vi "GUI_Cameras.vi"() -> ()   [LabVIEW 2009]
panel:
  out "Array":string[](array[string])
  out "Class Name":string
  out "appended array":refnum<vi>[](array[refnum])
  out "array":string[][](array[string])
  in  "Data String":string
  in  "time to wait":i32=100
  out "block device port":bool
  out "block slow port":bool
  out "new Slow Data":bool
  out "new Device Data":bool
  in  "Tab Control 2":enum32{"debug", "plain", "plain 2"}(tab)
  out "message from device":string
  out "data out 2":string
  out "error out 3":errorcluster
  in  "after substring 3":string
  out "settings 2":string[][](array[string])=[["no error", ">>on"]]
  out "after substring 2":string="no error,>>on"
  in  "Tab Control":enum32{"Main", "Network settings", "internal"}(tab)
  in  "getSettings":bool
  in  "setTrigger":bool
  in  "String":string="subscribe>>image"
  in  "sent":bool
  in  "setSave":bool
  out "save":bool
  in  "setExposure":dbl=2.0
  out "exposure":dbl=2.0
  out "value":string
  out "trigger":bool
  out "Image Pixels (U8) 5":u8[][](graph)
  out "gain":dbl=2.0
  in  "setGain":dbl=2.0
  in  "local Port":u16=61557
  in  "Remote Host":string="192.168.10.156"
  in  "port or service name":u16=65533
  in  "timeout ms (100)":i32=500
  out "fast ID":refnum<k16>
  out "slow ID":refnum<k16>
  out "error out":errorcluster
  in  "stop":bool
  # "61525"
  # "65535"
  # "61533"
  # "localhost"
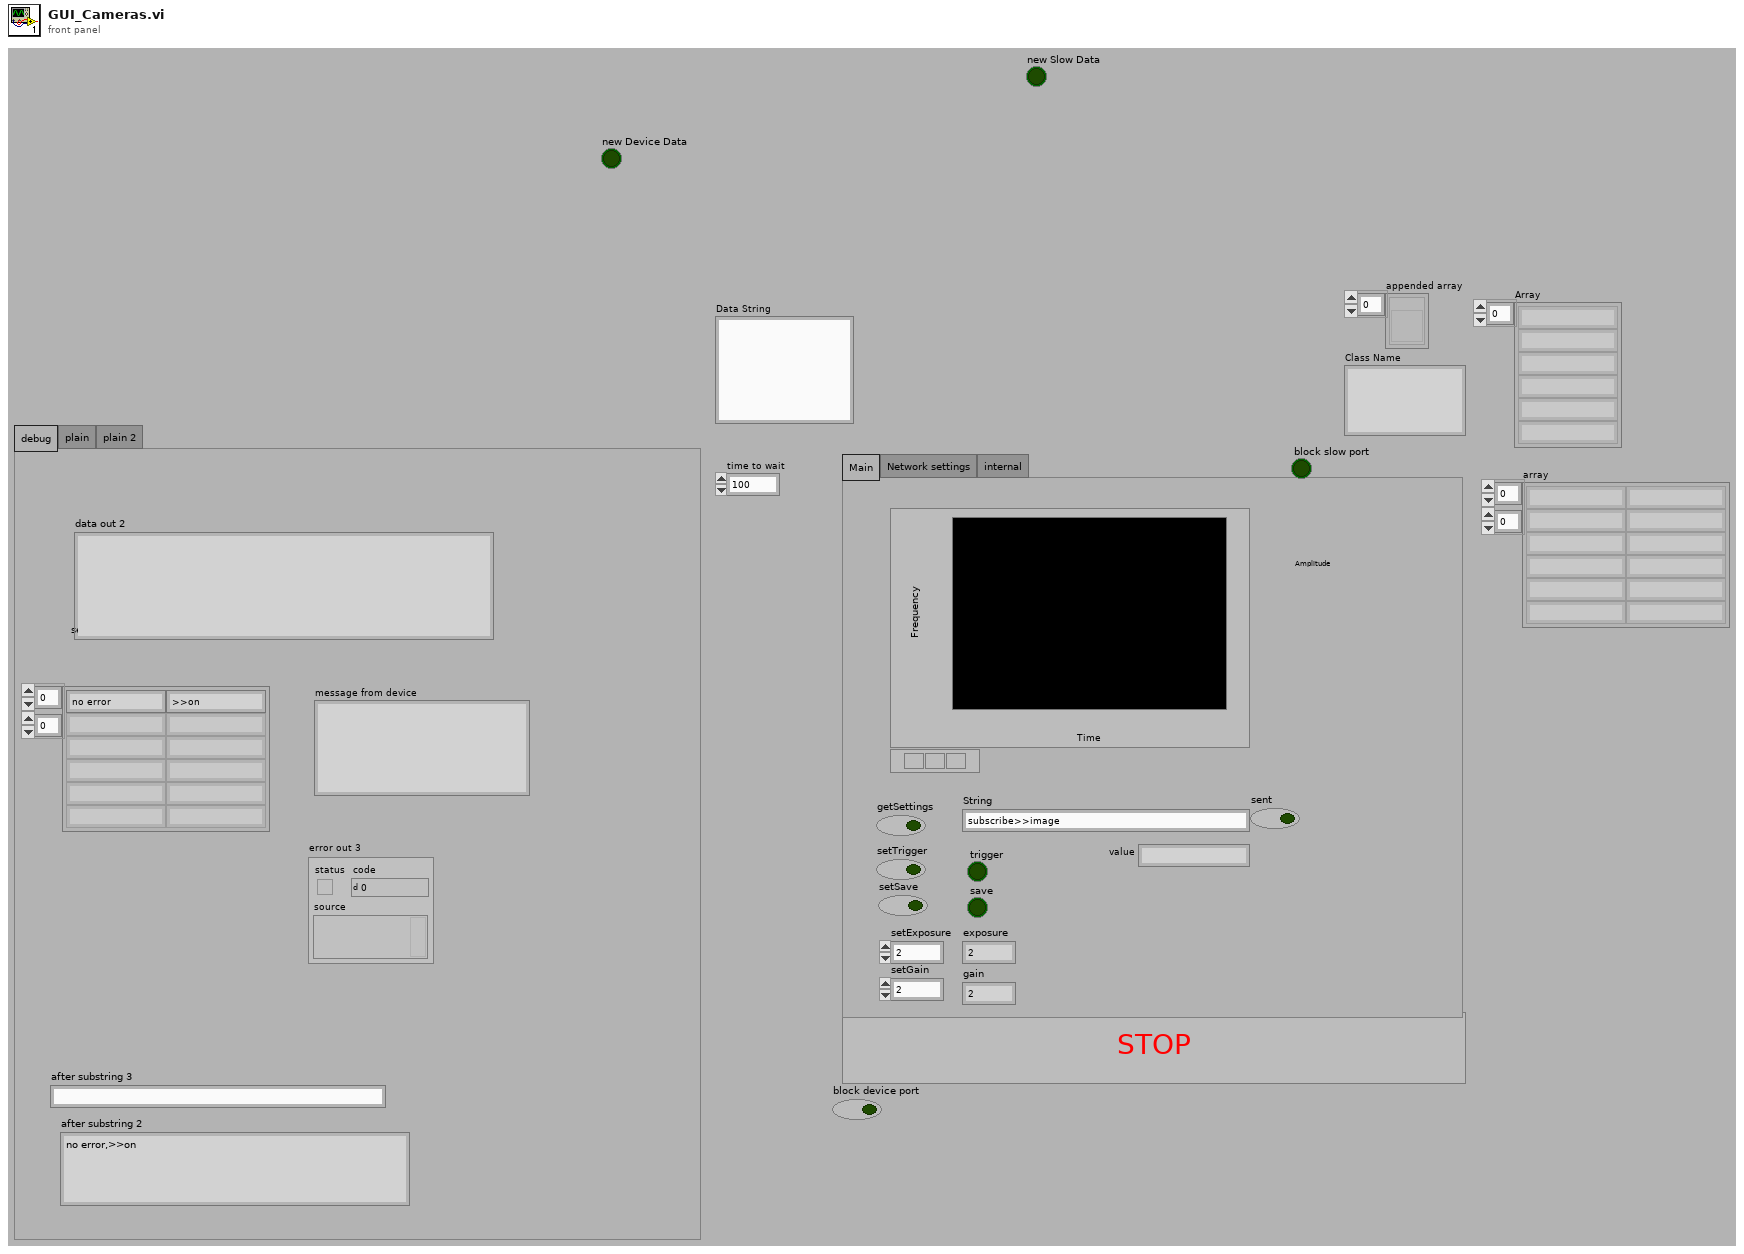
[diagram p1: front panel]
types:
  T1 = typedef "Image Type" = u32
  T2 = typedef "IMAQ Image.ctl" = refnum<image>
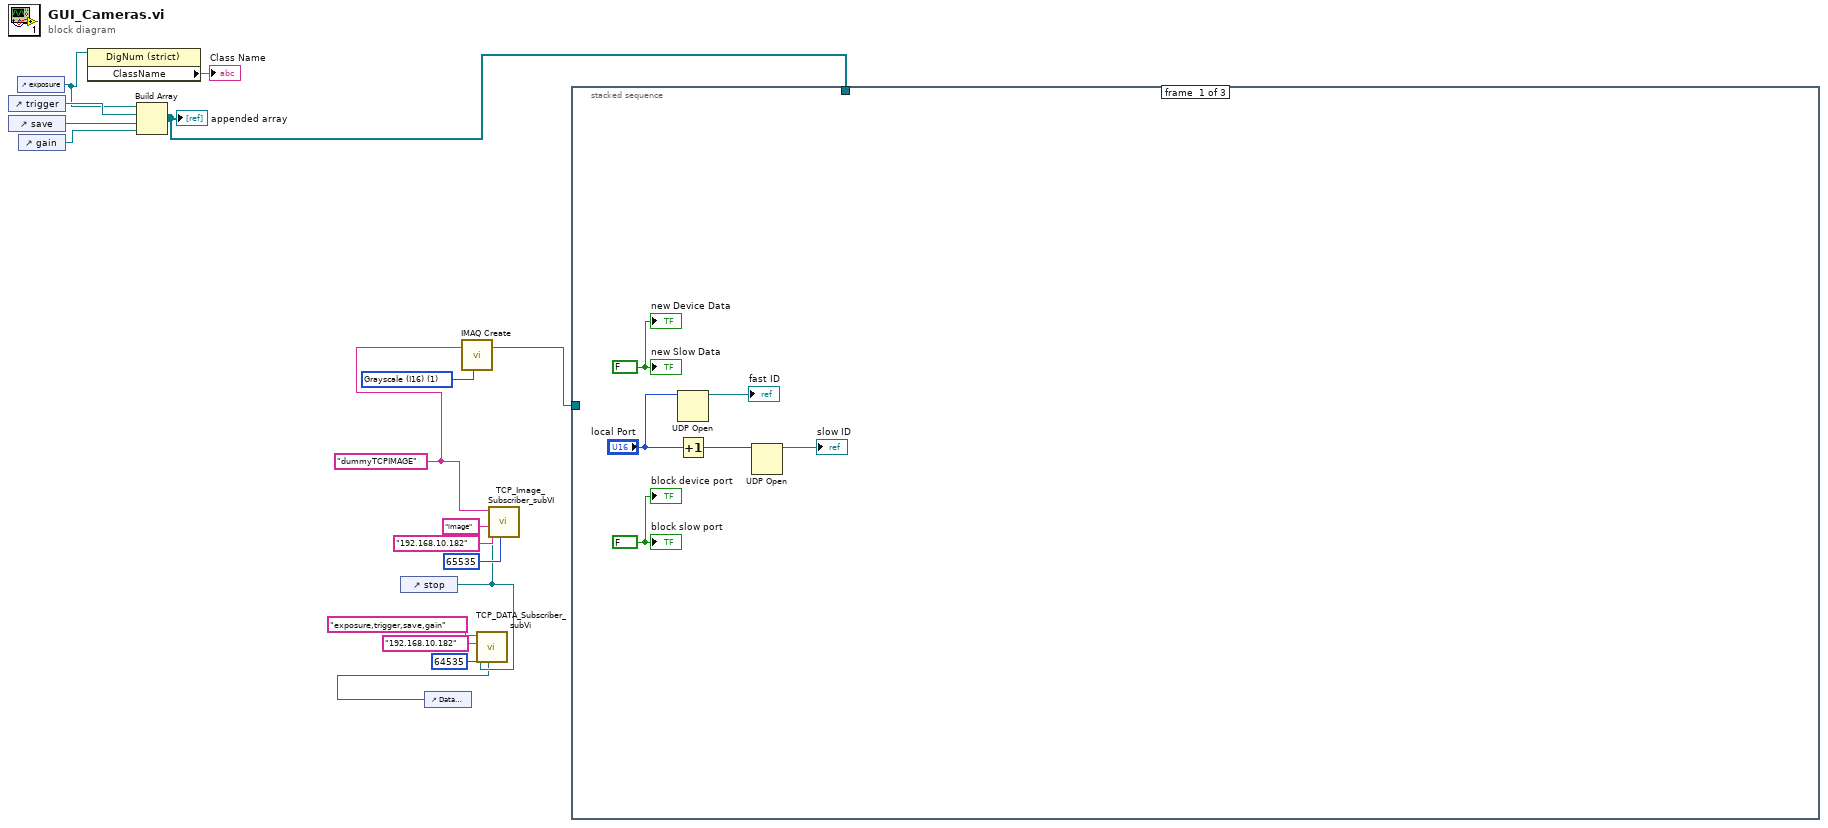
[diagram p0: block diagram]
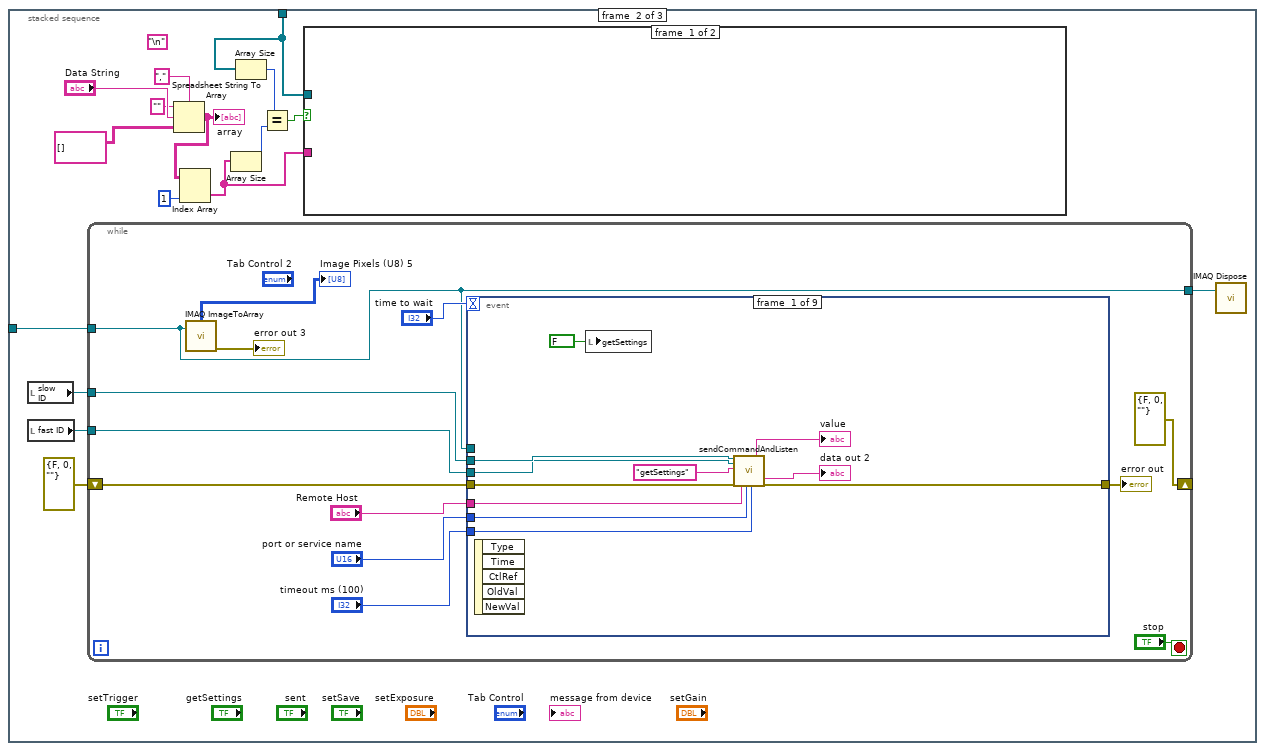
[diagram p2: hidden frame]
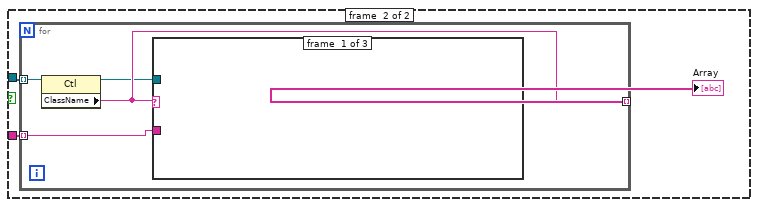
[diagram p3: hidden frame]
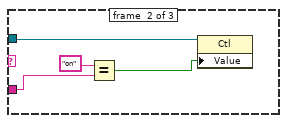
[diagram p4: hidden frame]
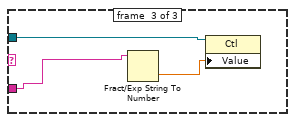
[diagram p5: hidden frame]
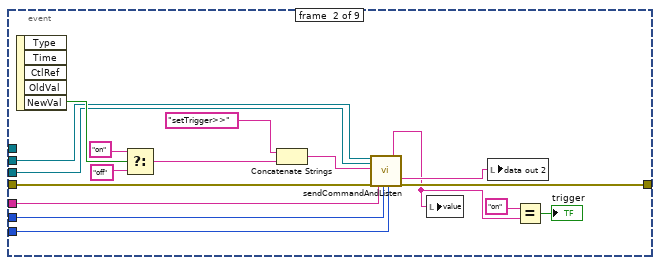
[diagram p6: hidden frame]
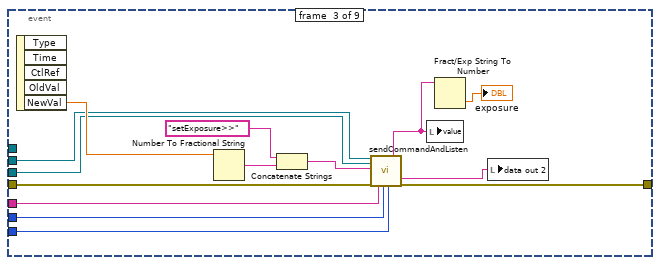
[diagram p7: hidden frame]
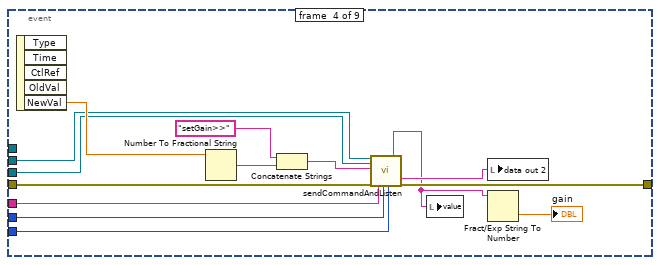
[diagram p8: hidden frame]
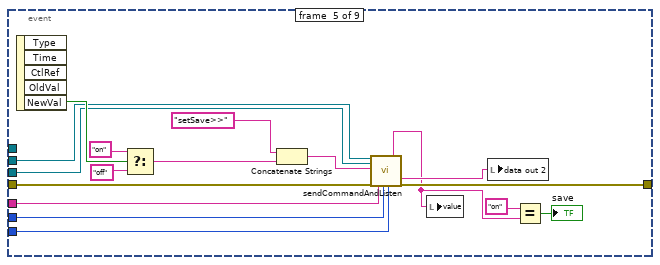
[diagram p9: hidden frame]
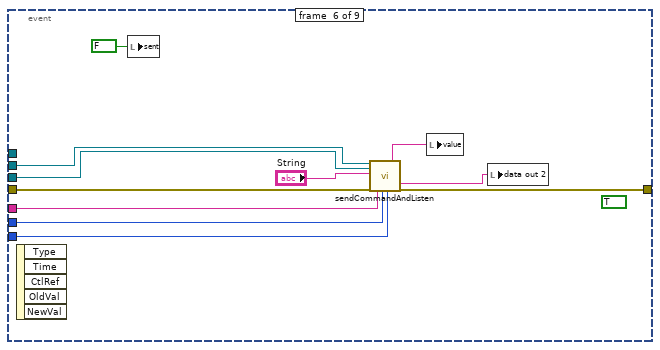
[diagram p10: hidden frame]
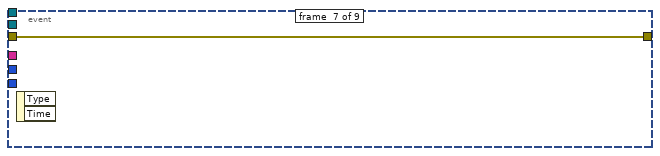
[diagram p11: hidden frame]
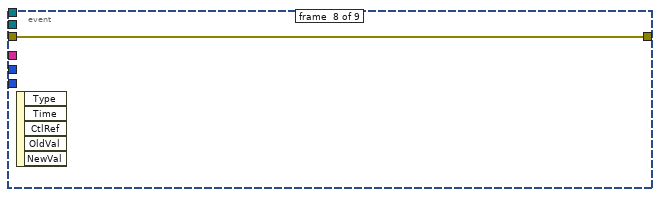
[diagram p12: hidden frame]
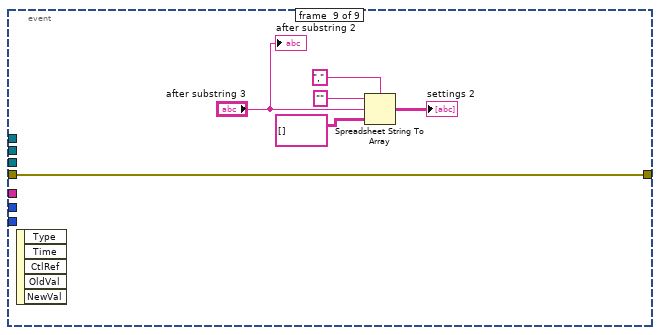
[diagram p13: hidden frame]
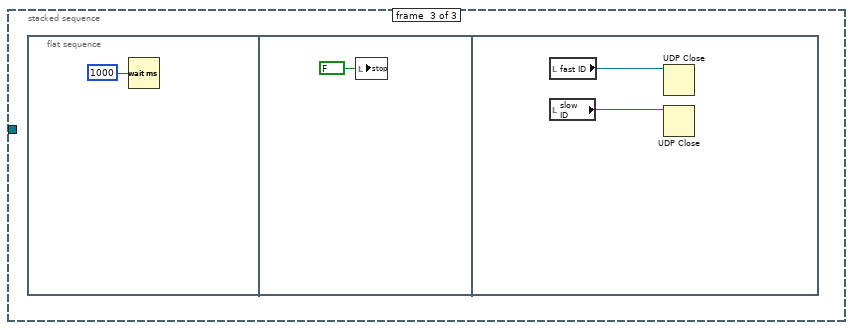
[diagram p14: hidden frame]
diagram:
  w12 = "dummyTCPIMAGE" ("Image Name")
  w17 = T1 1 items=["Grayscale (U8)", "Grayscale (I16)", "Grayscale (SGL)", "Complex (CSG)", "RGB (U32)", "HSL (U32)", "RGB (U64)", "Grayscale (U16)"] ("Image Type")
  n1 = control-ref of="trigger"() -> (w6:refnum<vi>)
  n2 = control-ref of="save"() -> (w5:refnum<vi>)
  n3 = control-ref of="exposure"() -> (w3:refnum<vi>)
  n4 = control-ref of="gain"() -> (w4:refnum<vi>)
  n5 = property class="DigNum (strict)"(reference=w3) -> ("ClassName"=→"Class Name":string)  [unwired: 1 in, 2 out]
  n6 = Build Array(w3, w6, w5, w4) -> (w1:refnum<vi>[])
  "appended array" <- w1
  n7 = control-ref of="stop"() -> (w8:refnum<vi>)
  n8 = control-ref of="Data String"() -> (w7:refnum<vi>)
  n9 = call "IMAQ Create"("Image Name"=w12, "Image Type"=w17) -> ("New Image"=w16:T2)  [unwired: 3 in, 1 out]
  n10 = call "TCP_DATA_Subscriber_subVi.vi"("data String"=w7, "stop 2"=w8, "Port"=u16 64535, "Machine"="192.168.10.182", "Subscriber list"="exposure,trigger,save,gain") -> ()  [unwired: 7 in]
  n11 = call "TCP_Image_Subscriber_subVI.vi"("Port"=u16 65535, "STOP"=w8, "Machine"="192.168.10.182", "subscriber list"="image", "Image Name"=w12) -> ()  [unwired: 7 in]
  n12 = stacked-sequence {
    tunnel: w16 -> [_ w36 _]
    tunnel: w1 -> [_ w30 _]
    frame #0 {
      w18 = FALSE ("new Device Data")
      w19 = FALSE
      n13 = UDP Open(11:"local Port") -> (port=→"fast ID":refnum<k16>)  [unwired: 4 in, 2 out]
      n14 = Increment(x="local Port") -> (x+1=w21:u16)
      n15 = UDP Open(11:w21) -> (port=→"slow ID":refnum<k16>)  [unwired: 4 in, 2 out]
      "block device port" <- w19
      "block slow port" <- w19
      "new Device Data" <- w18
      "new Slow Data" <- w18
    }
    frame #1 {
      (unwired) "\n"
      n16 = local read "slow ID"() -> (w37:refnum<k16>)
      n17 = local read "fast ID"() -> (w38:refnum<k16>)
      n18 = while {
        tunnel: w38 -> [w65]
        shift-right: [errorcluster {"status"=FALSE, "code"=0, "source"=""} ("error out")] -> _
        shift-left: errorcluster {"status"=FALSE, "code"=0, "source"=""} ("error out") -> [w63]
        tunnel: w37 -> [w57]
        tunnel: w36 -> [w54]
        tunnel: [w54] -> w35
        stop <- "stop" stop-if-true
        n19 = call "IMAQ ImageToArray"("Image"=w54) -> ("error out"=→"error out 3":errorcluster, "Image Pixels (U8)"=→"Image Pixels (U8) 5":u8[][])  [unwired: 3 in, 3 out]
        n20 = event shown="[2] \"setExposure\": Value Change" {
          selector: _ -> [_ _ _ _ _ _ _ _ _]
          dyn-events: _ -> [_ _ _ _ _ _ _ _ _]
          timeout: "time to wait" -> [_ _ _ _ _ _ _ _ _]
          tunnel: w65 -> [w74 w84 w103 w117 w132 w147 _ _ _]
          tunnel: [w72 w82 w101 w115 w129 w145 w151 w152 w158] -> w64
          tunnel: w63 -> [w73 w83 w102 w116 w130 w146 w151 w152 w158]
          tunnel: "Remote Host" -> [w71 w87 w99 w113 w133 w144 _ _ _]
          tunnel: "port or service name" -> [w70 w88 w98 w112 w128 w143 _ _ _]
          tunnel: "timeout ms (100)" -> [w69 w89 w97 w111 w127 w142 _ _ _]
          tunnel: w57 -> [w75 w85 w104 w118 w131 w148 _ _ _]
          tunnel: w54 -> [_ _ _ _ _ _ _ _ _]
          event #0 {
            n21 = event-data() -> ()  [unwired: 1 in, 5 out]
            n22 = local write "getSettings"(FALSE ("getSettings")) -> ()
            n23 = call "sendCommandAndListen.vi"("ID slow"=w75, "ID fast"=w74, "command in"="getSettings" ("data in"), "error in"=w73, "Remote Host"=w71, "port or service name"=w70, "timeout ms (100)"=w69) -> ("value"=→"value":string, "data out"=→"data out 2":string, "error out"=w72:errorcluster)  [unwired: 7 in, 3 out]
          }
          event #1 {
            n24 = event-data() -> ("NewVal"=w94:bool)  [unwired: 1 in, 4 out]
            n25 = Select(t="on", s=w94, f="off") -> (s? t:f=w90:string)
            n26 = Concatenate Strings("setTrigger>>" ("data in"), w90) -> (w86:string)
            n27 = call "sendCommandAndListen.vi"("ID slow"=w85, "ID fast"=w84, "command in"=w86, "error in"=w83, "Remote Host"=w87, "port or service name"=w88, "timeout ms (100)"=w89) -> ("value"=w79:string, "data out"=w81:string, "error out"=w82:errorcluster)  [unwired: 7 in, 3 out]
            n28 = local write "value"(w79) -> ()
            n29 = local write "data out 2"(w81) -> ()
            n30 = Equal?(x="on", y=w79) -> (x = y?=→"trigger":bool)
          }
          event #2 {
            n31 = event-data() -> ("NewVal"=w106:dbl)  [unwired: 1 in, 4 out]
            n32 = Number To Fractional String(number=w106) -> (F-format string=w107:string)  [unwired: 3 in]
            n33 = Concatenate Strings("setExposure>>" ("data in"), w107) -> (w105:string)
            n34 = call "sendCommandAndListen.vi"("ID slow"=w104, "ID fast"=w103, "command in"=w105, "error in"=w102, "Remote Host"=w99, "port or service name"=w98, "timeout ms (100)"=w97) -> ("value"=w96:string, "data out"=w100:string, "error out"=w101:errorcluster)  [unwired: 7 in, 3 out]
            n35 = local write "value"(w96) -> ()
            n36 = Fract/Exp String To Number(string=w96) -> (number=→"exposure":dbl)  [unwired: 3 in, 1 out]
            n37 = local write "data out 2"(w100) -> ()
          }
          event #3 {
            n38 = event-data() -> ("NewVal"=w120:dbl)  [unwired: 1 in, 4 out]
            n39 = Number To Fractional String(number=w120) -> (F-format string=w121:string)  [unwired: 3 in]
            n40 = Concatenate Strings("setGain>>" ("data in"), w121) -> (w119:string)
            n41 = call "sendCommandAndListen.vi"("ID slow"=w118, "ID fast"=w117, "command in"=w119, "error in"=w116, "Remote Host"=w113, "port or service name"=w112, "timeout ms (100)"=w111) -> ("value"=w110:string, "data out"=w114:string, "error out"=w115:errorcluster)  [unwired: 7 in, 3 out]
            n42 = local write "value"(w110) -> ()
            n43 = local write "data out 2"(w114) -> ()
            n44 = Fract/Exp String To Number(string=w110) -> (number=→"gain":dbl)  [unwired: 3 in, 1 out]
          }
          event #4 {
            n45 = event-data() -> ("NewVal"=w139:bool)  [unwired: 1 in, 4 out]
            n46 = Select(t="on", s=w139, f="off") -> (s? t:f=w135:string)
            n47 = Concatenate Strings("setSave>>" ("data in"), w135) -> (w134:string)
            n48 = call "sendCommandAndListen.vi"("ID slow"=w131, "ID fast"=w132, "command in"=w134, "error in"=w130, "Remote Host"=w133, "port or service name"=w128, "timeout ms (100)"=w127) -> ("value"=w125:string, "data out"=w126:string, "error out"=w129:errorcluster)  [unwired: 7 in, 3 out]
            n49 = local write "value"(w125) -> ()
            n50 = local write "data out 2"(w126) -> ()
            n51 = Equal?(x="on", y=w125) -> (x = y?=→"save":bool)
          }
          event #5 {
            (unwired) TRUE ("Boolean")
            n52 = event-data() -> ()  [unwired: 1 in, 5 out]
            n53 = local write "sent"(FALSE ("sent")) -> ()
            n54 = call "sendCommandAndListen.vi"("ID slow"=w148, "ID fast"=w147, "command in"="String", "error in"=w146, "Remote Host"=w144, "port or service name"=w143, "timeout ms (100)"=w142) -> ("value"=w140:string, "data out"=w141:string, "error out"=w145:errorcluster)  [unwired: 7 in, 3 out]
            n55 = local write "value"(w140) -> ()
            n56 = local write "data out 2"(w141) -> ()
          }
          event #6 {
            n57 = event-data() -> ()  [unwired: 1 in, 2 out]
          }
          event #7 {
            n58 = event-data() -> ()  [unwired: 1 in, 5 out]
          }
          event #8 {
            n59 = event-data() -> ()  [unwired: 1 in, 5 out]
            n60 = Spreadsheet String To Array(delimiter (Tab)=",", format string="", spreadsheet string="after substring 3", array type (2D Dbl)=string[][] []) -> (array=→"settings 2":string[][])
            "after substring 2" <- "after substring 3"
          }
        }
        "error out" <- w64
      }
      n61 = Spreadsheet String To Array(delimiter (Tab)=",", format string="", spreadsheet string="Data String", array type (2D Dbl)=string[][] []) -> (array=w27:string[][])
      "array" <- w27
      n62 = Index Array(array=w27, index (col)=1 ("disabled index (col)")) -> (element=w24:string[])  [unwired: 1 in]
      n63 = Array Size(array=w24) -> (size(s)=w29:i32)
      n64 = Array Size(array=w30) -> (size(s)=w28:i32)
      n65 = Equal?(x=w28, y=w29) -> (x = y?=w25:bool)
      n66 = case shown="True" w25 {
        tunnel: w30 -> [_ w41]
        tunnel: w24 -> [_ w40]
        frame #0 {
        }
        frame #1 {
          n67 = for {
            tunnel: w41 -> [w46] mode=indexing
            tunnel: [w45] -> w42 mode=indexing
            tunnel: w40 -> [w44] mode=indexing
            n68 = property class="Ctl"(reference=w46) -> (reference out=w43:refnum<vi>, "ClassName"=w45:string)  [unwired: 1 in, 1 out]
            n69 = case shown="\"Digital\"" w45 {
              tunnel: w44 -> [_ w49 w51]
              tunnel: w43 -> [_ w48 w52]
              frame #0 {
              }
              frame #1 {
                n70 = Equal?(x="on", y=w49) -> (x = y?=w47:bool)
                n71 = property class="Ctl"(reference=w48, "Value"=w47) -> ()  [unwired: 1 in, 2 out]
              }
              frame #2 {
                n72 = Fract/Exp String To Number(string=w51) -> (number=w53:dbl)  [unwired: 3 in, 1 out]
                n73 = property class="Ctl"(reference=w52, "Value"=w53) -> ()  [unwired: 1 in, 2 out]
              }
            }
          }
          "Array" <- w42
        }
      }
      n74 = call "IMAQ Dispose"("Image"=w35) -> ()  [unwired: 5 in, 1 out]
    }
    frame #2 {
      n75 = flat-sequence {
        frame #0 {
          n76 = Wait (ms)(milliseconds to wait=u32 1000) -> ()  [unwired: 1 out]
        }
        frame #1 {
          n77 = local write "stop"(FALSE ("stop")) -> ()
        }
        frame #2 {
          n78 = local read "fast ID"() -> (w161:refnum<k16>)
          n79 = local read "slow ID"() -> (w162:refnum<k16>)
          n80 = UDP Close(connection ID=w161) -> ()  [unwired: 1 in, 2 out]
          n81 = UDP Close(connection ID=w162) -> ()  [unwired: 1 in, 2 out]
        }
      }
    }
  }
